vi "Send Get Pending IMatch Responses.vi"(7 "Message Priority (Normal)":T1=enum."Normal", 8 "error in (no error)":errorcluster, 11 "Message Enqueuer":refnum<class "Message Enqueuer.lvclass">) -> (0 "error out":errorcluster, 3 "Message Enqueuer out":refnum<class "Message Enqueuer.lvclass">)   [LabVIEW 2020, in "CANopen.lvlib" / "Response Matcher.lvlib" / "Get Pending IMatch Responses Reply Msg.lvclass"]
doc: "This VI sends the message to an actor."
uses:
  Get Pending IMatch Responses Reply Msg.lvclass
  Get Pending IMatch Responses Reply Msg.lvclass/Get Pending IMatch Responses Reply Msg.ctl
  C:/Program Files/National Instruments/LabVIEW 2026/vi.lib/ActorFramework/Specialty Messages/Reply Msg/Reply Msg.lvclass
  C:/Program Files/National Instruments/LabVIEW 2026/vi.lib/ActorFramework/Message/Message.lvclass
  D:/git/CANopen-LabVIEW/source/Response Matcher/Response Matcher Messages/Get Pending IMatch Responses Msg/Get Pending IMatch Responses Reply Msg.lvclass
  <vilib>/ActorFramework/Message Enqueuer/Message Enqueuer.lvclass
  <vilib>/ActorFramework/Message Enqueuer/Message Priority.ctl
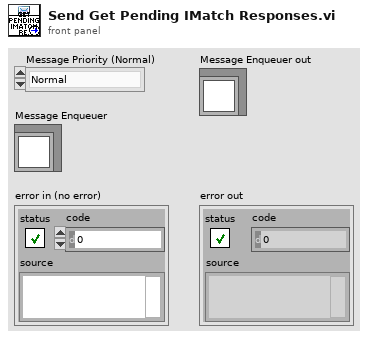
[diagram p1: front panel]
types:
  T1 = typedef "Actor Framework.lvlib/Message Enqueuer.lvclass/Message Priority.ctl" = enum16{"Low", "Normal", "High"}
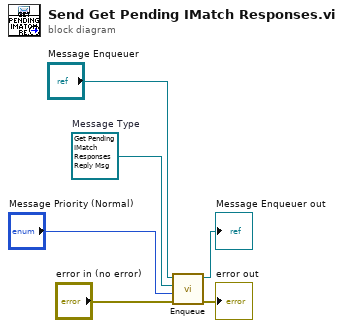
[diagram p0: block diagram]
diagram:
  w1 = refnum<class "Get Pending IMatch Responses Reply Msg.lvclass"> refnum  # Message Type
  n1 = call <vilib>:"Enqueue.vi"("error in (no error)"="error in (no error)", "Message Priority (Normal)"="Message Priority (Normal)", "Message"=w1, "Message Enqueuer in"="Message Enqueuer") -> ("error out"=→"error out":errorcluster, "Message Enqueuer out"=→"Message Enqueuer out":refnum<class "Message Enqueuer.lvclass">)  [unwired: 6 in]
